vi "DoExecute.vi"(0 "reference in":refnum<class "Executer.lvclass">, 1 "Class":string, 2 "Method":string, 3 "Inputs":variant[](array[variant]), 5 "error in (no error)":errorcluster) -> (14 "reference out":refnum<class "Executer.lvclass">, 17 "Outputs":variant[](array[variant]), 19 "error out":errorcluster)   [LabVIEW 2018, in "Executer.lvclass"]
doc: "Executes the VI mentioned at the inputs with all the data, and returns the output of that VI. \nTake in mind the executing VI error is merged on the error wire."
uses:
  Executer.lvclass
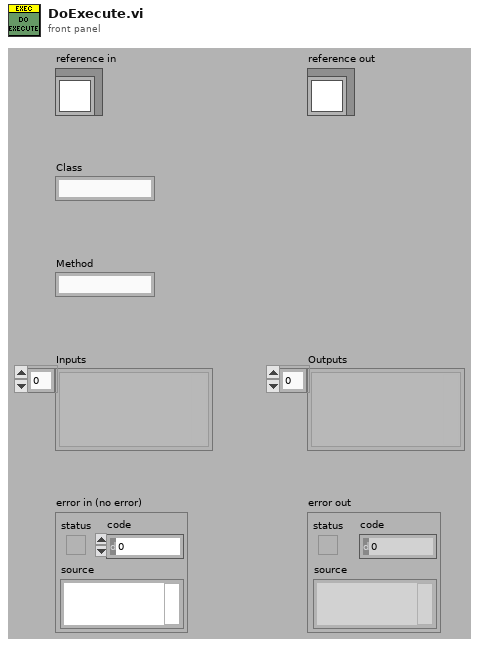
[diagram p1: front panel]
types:
  T1 = typedef "Executer.lvclass/MethodExecutionInfo.ctl" = cluster{"viRef":refnum<vi>, "MethodName":string, "ControlIndices":i32[], "ClassInIndex":i32, "IndicatorIndices":i32[], "ErrorOutIndex":i32, "ControlTypes":variant[]}
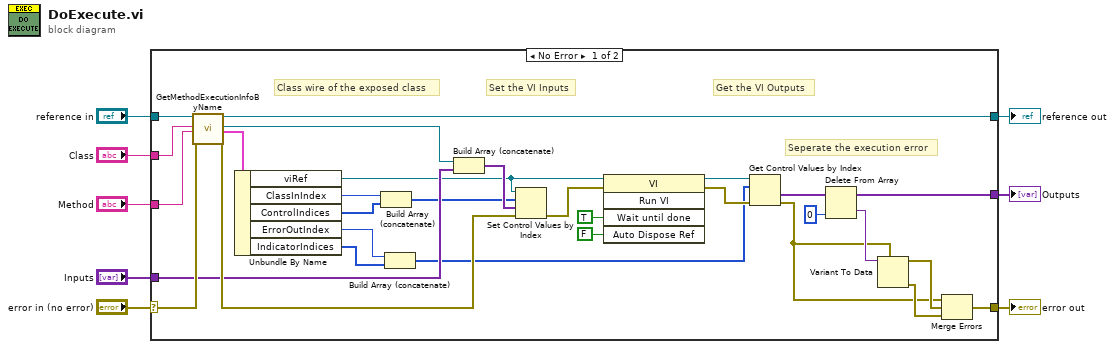
[diagram p0: block diagram]
diagram:
  n1 = case shown="No Error" "error in (no error)" {
    selector: "error in (no error)" -> [w37 w40]
    tunnel: [w15 w40] -> w7
    tunnel: [w34 w39] -> w5
    tunnel: "reference in" -> [w35 w39]
    tunnel: "Class" -> [w33 _]
    tunnel: "Method" -> [w32 _]
    tunnel: [w11 _] -> w2
    tunnel: "Inputs" -> [w29 _]
    frame No Error {
      # "Seperate the execution error"
      # "Get the VI Outputs"
      # "Set the VI Inputs"
      # "Class wire of the exposed class"
      n2 = call "GetMethodExecutionInfoByName.vi"("Executer in"=w35, "Class in"=w33, "Method"=w32, "error in (no error)"=w37) -> ("Executer out"=w34:refnum<class "Executer.lvclass">, "Class"=w30:refnum<class>, "Method"=w31:T1, "error out"=w36:errorcluster)  [unwired: 12 in]
      n3 = Unbundle By Name(w31) -> ("viRef"=w9:refnum<vi>, "ClassInIndex"=w28:i32, "ControlIndices"=w27:i32[], "ErrorOutIndex"=w17:i32, "IndicatorIndices"=w13:i32[])
      n4 = Build Array (concatenate)(w28, w27) -> (w20:i32[])
      n5 = Build Array (concatenate)(w17, w13) -> (w19:i32[])
      n6 = Build Array (concatenate)(w30, w29) -> (w24:variant[])
      n7 = Set Control Values by Index(0:w9, 1:w20, 2:w24, 3:w36) -> (11:w21:errorcluster)
      n8 = invoke class="VI" method="Run VI"(reference=w9, error in=w21, "Wait until done"=TRUE ("Wait Until Done"), "Auto Dispose Ref"=FALSE ("Auto Dispose Reference")) -> (reference out=w16:refnum<vi>, error out=w38:errorcluster)  [unwired: 1 in, 3 out]
      n9 = Get Control Values by Index(0:w16, 1:w19, 3:w38) -> (10:w23:variant[], 11:w10:errorcluster)
      n10 = Delete From Array(array=w23, index=0) -> (deleted portion=w22:variant, array with subset deleted=w11:variant[])  [unwired: 1 in]
      n11 = Variant To Data(type=w10, Variant=w22) -> (data=w18:errorcluster, error out=w14:errorcluster)  [unwired: 1 in]
      n12 = Merge Errors(w10, w18, w14) -> (w15:errorcluster)
    }
    frame Error {
    }
  }
  "error out" <- w7
  "reference out" <- w5
  "Outputs" <- w2
